vi "Element Type.vi"(11 "Sequencing Control in":refnum<class "Sequencing Control.lvclass">) -> (2 "Element Type":string)   [LabVIEW 2020, in "VolatusSeqGUI.lvlib" / "Sequencing Control.lvclass"]
uses:
  Sequencing Control.lvclass
  Sequencing Control.lvclass/Sequencing Control.ctl
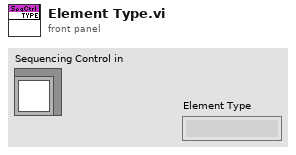
[diagram p1: front panel]
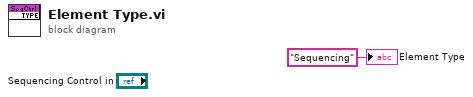
[diagram p0: block diagram]
diagram:
  "Element Type" <- "Sequencing" ("Element Type")
